vi "Write Data.vi"(8 "error in (no error)":errorcluster, 10 "AbstractData.lvclass":refnum<class "AbstractData.lvclass">, 11 "Data Msg in":refnum<class "Data Msg.lvclass">) -> (0 "error out":errorcluster, 3 "Data Msg out":refnum<class "Data Msg.lvclass">)   [LabVIEW 2014, in "Data Msg.lvclass"]
uses:
  Data Msg.lvclass
  Data/AbstractData/AbstractData.lvclass
  Data Msg.lvclass/Data Msg.ctl
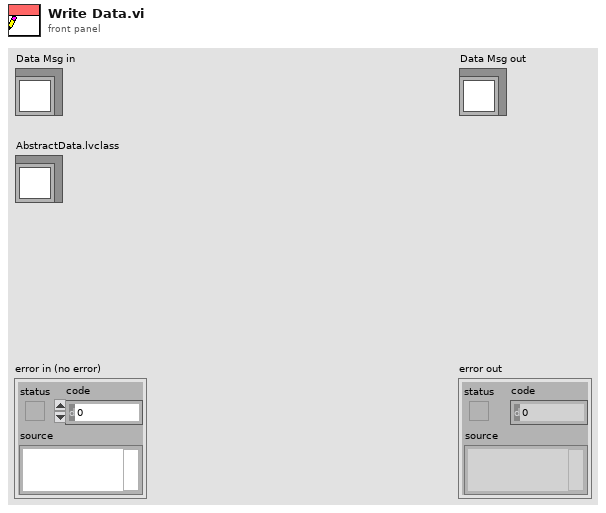
[diagram p1: front panel]
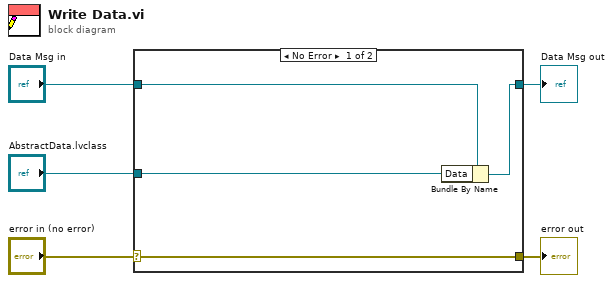
[diagram p0: block diagram]
diagram:
  n1 = case shown="No Error" "error in (no error)" {
    selector: "error in (no error)" -> [w9 w10]
    tunnel: [w9 w10] -> w4
    tunnel: [w7 w11] -> w2
    tunnel: "Data Msg in" -> [w8 w11]
    tunnel: "AbstractData.lvclass" -> [w6 _]
    frame No Error {
      n2 = Bundle By Name(cluster=w8, "Data"=w6) -> (w7:refnum<class "Data Msg.lvclass">)
    }
    frame Error {
    }
  }
  "error out" <- w4
  "Data Msg out" <- w2
